vi "FGV CalGas.vi"(6 "Aktionen":T8, 7 "Analysator Auswahl":T1 {"Analysator Auswahl 12" items=["----"=100, "FT-IR"=0, "TEST"=1]; "Analysator Auswahl 11" items=["----"=100, "FT-IR"=0, "TEST"=1]; "Analysator Auswahl 10" items=["----"=100, "FT-IR"=0, "TEST"=1]; "Analysator Auswahl 9" items=["----"=100, "FT-IR"=0, "TEST"=1]; "Analysator Auswahl 8" items=["----"=100, "FT-IR"=0, "TEST"=1]; "Analysator Auswahl 7" items=["----"=100, "FT-IR"=0, "TEST"=1]; "Analysator Auswahl 6" items=["----"=100, "FT-IR"=0, "TEST"=1]; "Analysator Auswahl 5" items=["----"=100, "FT-IR"=0, "TEST"=1]; "Analysator Auswahl 4" items=["----"=100, "FT-IR"=0, "TEST"=1]; "Analysator Auswahl 3" items=["----"=100, "FT-IR"=0, "TEST"=1]; "Analysator Auswahl 2" items=["----"=100, "FT-IR"=0, "TEST"=1]; "Analysator Auswahl" items=["----"=100, "FT-IR"=0, "PMA"=1]}, 10 "Aufschaltung CalGas":T4 {"Kalibriergas" items=["Stickstoff", "---", "---", "NOx lo", "NOx hi", "---", "CO2", "CO", "---", "O2", "---", "HC", "---"]}, 11 "Def.CalGas neu":T9 {"Messbereiche"."Messbereich 12" items=["0-100ppm", "0-1000ppm", "0-5000ppm"]; "Messbereiche"."Messbereich 11" items=["0-100ppm", "0-1000ppm", "0-5000ppm"]; "Messbereiche"."Messbereich 10" items=["0-100ppm", "0-1000ppm", "0-5000ppm"]; "Messbereiche"."Messbereich 9" items=["0-100ppm", "0-1000ppm", "0-5000ppm"]; "Messbereiche"."Messbereich 8" items=["0-100ppm", "0-1000ppm", "0-5000ppm"]; "Messbereiche"."Messbereich 7" items=["0-100ppm", "0-1000ppm", "0-5000ppm"]; "Messbereiche"."Messbereich 6" items=["0-100ppm", "0-1000ppm", "0-5000ppm"]; "Messbereiche"."Messbereich 5" items=["0-100ppm", "0-1000ppm", "0-5000ppm"]; "Messbereiche"."Messbereich 4" items=["0-100ppm", "0-1000ppm", "0-5000ppm"]; "Messbereiche"."Messbereich 3" items=["0-100ppm", "0-1000ppm", "0-5000ppm"]; "Messbereiche"."Messbereich 2" items=["0-100ppm", "0-1000ppm", "0-5000ppm"]; "Messbereiche"."Messbereich 1" items=["0-100ppm", "0-1000ppm", "0-5000ppm"]; "Einheit"."Einheit 12" items=["ppm", "%"]; "Einheit"."Einheit 11" items=["ppm", "%"]; "Einheit"."Einheit 10" items=["ppm", "%"]; "Einheit"."Einheit 9" items=["ppm", "%"]; "Einheit"."Einheit 8" items=["ppm", "%"]; "Einheit"."Einheit 7" items=["ppm", "%"]; "Einheit"."Einheit 6" items=["ppm", "%"]; "Einheit"."Einheit 5" items=["ppm", "%"]; "Einheit"."Einheit 4" items=["ppm", "%"]; "Einheit"."Einheit 3" items=["ppm", "%"]; "Einheit"."Einheit 2" items=["ppm", "%"]; "Einheit"."Einheit 1" items=["ppm", "%"]; "Werte 2"."Konzentration 12" format="%#_5g"; "Werte 2"."Konzentration 11" format="%#_5g"; "Werte 2"."Konzentration 10" format="%#_5g"; "Werte 2"."Konzentration 9" format="%#_5g"; "Werte 2"."Konzentration 8" format="%#_5g"; "Werte 2"."Konzentration 7" format="%#_5g"; "Werte 2"."Konzentration 6" format="%#_5g"; "Werte 2"."Konzentration 5" format="%#_5g"; "Werte 2"."Konzentration 4" format="%#_5g"; "Werte 2"."Konzentration 3" format="%#_5g"; "Werte 2"."Konzentration 2" format="%#_5g"; "Werte 2"."Konzentration 1" format="%#_5g"; "Werte"."Konzentration 12" format="%#_5g"; "Werte"."Konzentration 11" format="%#_5g"; "Werte"."Konzentration 10" format="%#_5g"; "Werte"."Konzentration 9" format="%#_5g"; "Werte"."Konzentration 8" format="%#_5g"; "Werte"."Konzentration 7" format="%#_5g"; "Werte"."Konzentration 6" format="%#_5g"; "Werte"."Konzentration 5" format="%#_5g"; "Werte"."Konzentration 4" format="%#_5g"; "Werte"."Konzentration 3" format="%#_5g"; "Werte"."Konzentration 2" format="%#_5g"; "Werte"."Konzentration 1" format="%#_5g"}) -> (0 "Konzentration 2":T3 format="%#_5g", 1 "Konzentration 1":T3 format="%#_5g", 2 "Aufschaltung CalGas":T4, 3 "Def.CalGas":T9 {"Messbereiche"."Messbereich 12" items=["0-100ppm", "0-1000ppm", "0-5000ppm"]; "Messbereiche"."Messbereich 11" items=["0-100ppm", "0-1000ppm", "0-5000ppm"]; "Messbereiche"."Messbereich 10" items=["0-100ppm", "0-1000ppm", "0-5000ppm"]; "Messbereiche"."Messbereich 9" items=["0-100ppm", "0-1000ppm", "0-5000ppm"]; "Messbereiche"."Messbereich 8" items=["0-100ppm", "0-1000ppm", "0-5000ppm"]; "Messbereiche"."Messbereich 7" items=["0-100ppm", "0-1000ppm", "0-5000ppm"]; "Messbereiche"."Messbereich 6" items=["0-100ppm", "0-1000ppm", "0-5000ppm"]; "Messbereiche"."Messbereich 5" items=["0-100ppm", "0-1000ppm", "0-5000ppm"]; "Messbereiche"."Messbereich 4" items=["0-100ppm", "0-1000ppm", "0-5000ppm"]; "Messbereiche"."Messbereich 3" items=["0-100ppm", "0-1000ppm", "0-5000ppm"]; "Messbereiche"."Messbereich 2" items=["0-100ppm", "0-1000ppm", "0-5000ppm"]; "Messbereiche"."Messbereich 1" items=["0-100ppm", "0-1000ppm", "0-5000ppm"]; "Einheit"."Einheit 12" items=["ppm", "%"]; "Einheit"."Einheit 11" items=["ppm", "%"]; "Einheit"."Einheit 10" items=["ppm", "%"]; "Einheit"."Einheit 9" items=["ppm", "%"]; "Einheit"."Einheit 8" items=["ppm", "%"]; "Einheit"."Einheit 7" items=["ppm", "%"]; "Einheit"."Einheit 6" items=["ppm", "%"]; "Einheit"."Einheit 5" items=["ppm", "%"]; "Einheit"."Einheit 4" items=["ppm", "%"]; "Einheit"."Einheit 3" items=["ppm", "%"]; "Einheit"."Einheit 2" items=["ppm", "%"]; "Einheit"."Einheit 1" items=["ppm", "%"]; "Werte 2"."Konzentration 12" format="%#_5g"; "Werte 2"."Konzentration 11" format="%#_5g"; "Werte 2"."Konzentration 10" format="%#_5g"; "Werte 2"."Konzentration 9" format="%#_5g"; "Werte 2"."Konzentration 8" format="%#_5g"; "Werte 2"."Konzentration 7" format="%#_5g"; "Werte 2"."Konzentration 6" format="%#_5g"; "Werte 2"."Konzentration 5" format="%#_5g"; "Werte 2"."Konzentration 4" format="%#_5g"; "Werte 2"."Konzentration 3" format="%#_5g"; "Werte 2"."Konzentration 2" format="%#_5g"; "Werte 2"."Konzentration 1" format="%#_5g"; "Werte"."Konzentration 12" format="%#_5g"; "Werte"."Konzentration 11" format="%#_5g"; "Werte"."Konzentration 10" format="%#_5g"; "Werte"."Konzentration 9" format="%#_5g"; "Werte"."Konzentration 8" format="%#_5g"; "Werte"."Konzentration 7" format="%#_5g"; "Werte"."Konzentration 6" format="%#_5g"; "Werte"."Konzentration 5" format="%#_5g"; "Werte"."Konzentration 4" format="%#_5g"; "Werte"."Konzentration 3" format="%#_5g"; "Werte"."Konzentration 2" format="%#_5g"; "Werte"."Konzentration 1" format="%#_5g"}, 5 "Analysator Auswahl":T1 {"Analysator Auswahl 12" items=["----"=100, "FT-IR"=0, "TEST"=1]; "Analysator Auswahl 11" items=["----"=100, "FT-IR"=0, "TEST"=1]; "Analysator Auswahl 10" items=["----"=100, "FT-IR"=0, "TEST"=1]; "Analysator Auswahl 9" items=["----"=100, "FT-IR"=0, "TEST"=1]; "Analysator Auswahl 8" items=["----"=100, "FT-IR"=0, "TEST"=1]; "Analysator Auswahl 7" items=["----"=100, "FT-IR"=0, "TEST"=1]; "Analysator Auswahl 6" items=["----"=100, "FT-IR"=0, "TEST"=1]; "Analysator Auswahl 5" items=["----"=100, "FT-IR"=0, "TEST"=1]; "Analysator Auswahl 4" items=["----"=100, "FT-IR"=0, "TEST"=1]; "Analysator Auswahl 3" items=["----"=100, "FT-IR"=0, "TEST"=1]; "Analysator Auswahl 2" items=["----"=100, "FT-IR"=0, "TEST"=1]; "Analysator Auswahl" items=["----"=100, "FT-IR"=0, "PMA"=1]})   [LabVIEW 2020, in "CalGas Aufschaltung.lvlib"]
uses:
  CalGas Aufschaltung.lvlib
  Definition CalGas Anzeige.ctl
  CalGas-Namen.ctl
  Visualisierungs Elemente/String - Eingabefeld.ctl
  CalGas-Werte.ctl
  Visualisierungs Elemente/Zahlen-Eingabefeld.ctl
  CalGas-Einheit.ctl
  Visualisierungs Elemente/Auswahlfeld.ctl
  CalGas-Messbereiche.ctl
  FGV CalGas Aktionen.ctl
  Aufschaltung CalGas.ctl
  Auswahl Aufschaltpunkt.ctl
  Auswahl Analysator.ctl
  Cluster Auswahl Analysator.ctl
  Analysator Auswahl.ctl
  Analysator Definition/FGV Analysator Definition Aktionen.ctl
  Allgemein/allgemeine Sub-VIs.lvlib
  Analysator Definition/Analysator Definition.lvlib
panel:
  # "Span 1"
  # "Span 2"
  # "Span 3"
  # "Span 4"
  # "Span 5"
  # "Span 6"
  # "Span 7"
  # "Span 8"
  # "Span 9"
  # "Span 10"
  # "Span 11"
  # "Span 12"
  # "Span 1"
  # "Span 2"
  # "Span 3"
  # "Span 4"
  # "Span 5"
  # "Span 6"
  # "Span 7"
  # "Span 8"
  # "Span 9"
  # "Span 10"
  # "Span 11"
  # "Span 12"
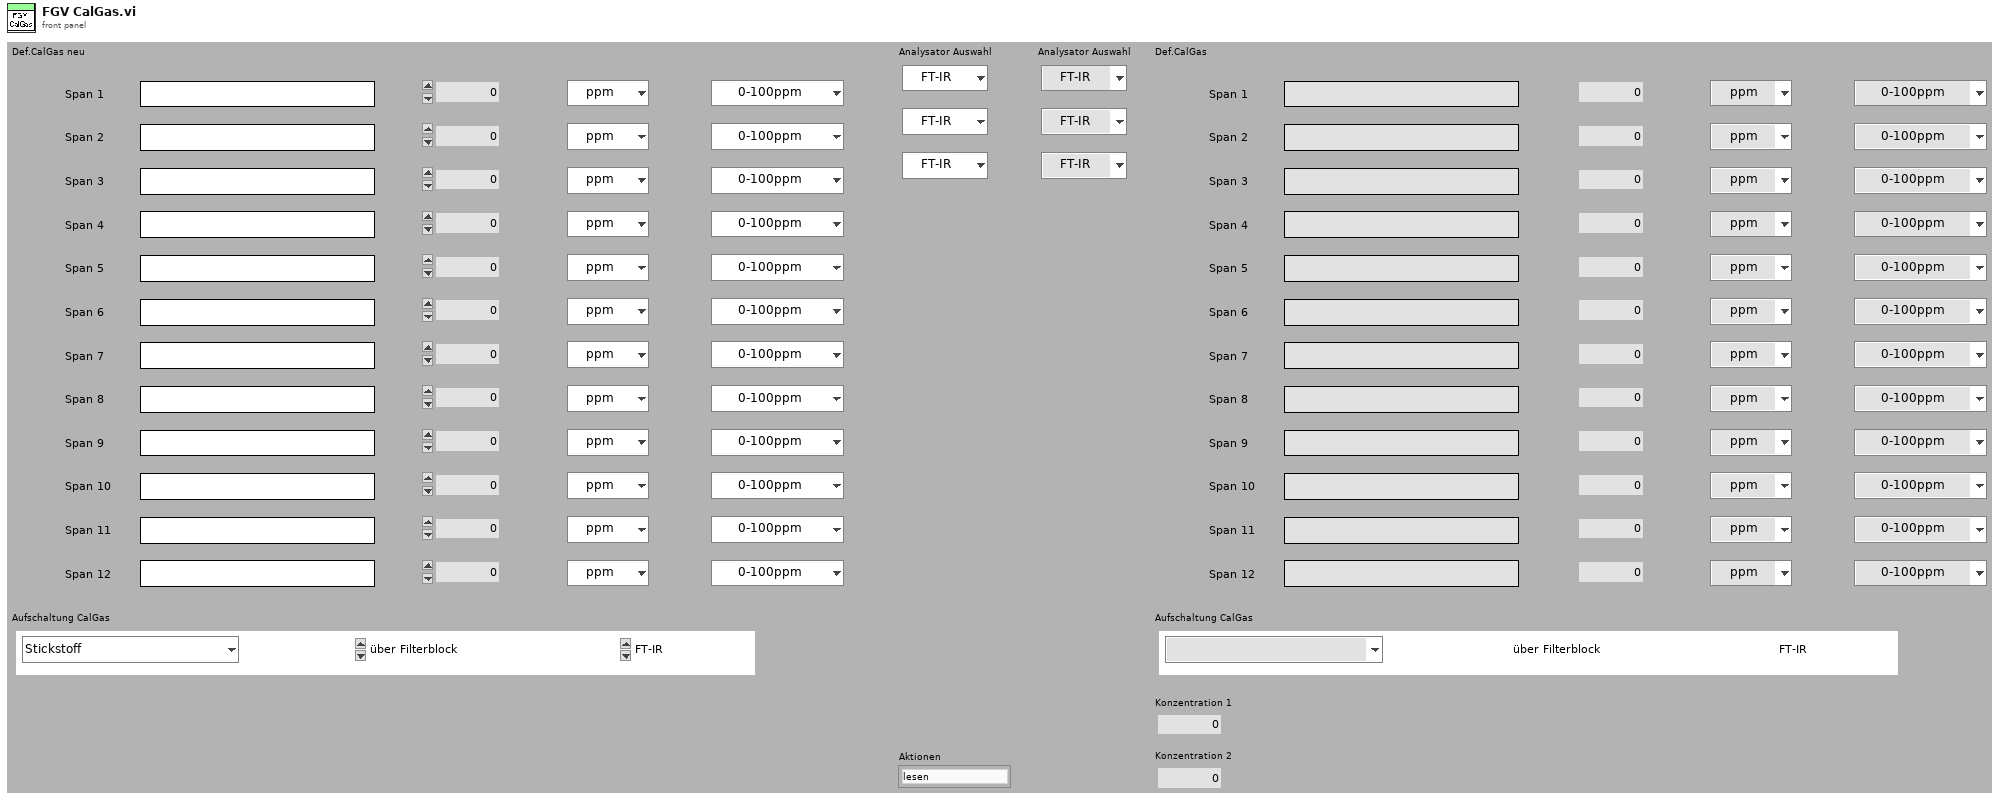
[diagram p1: front panel]
types:
  T1 = typedef "CalGas Aufschaltung.lvlib/Cluster Auswahl Analysator.ctl" = cluster{"Analysator Auswahl":T2, "Analysator Auswahl 2":T2, "Analysator Auswahl 3":T2, "Analysator Auswahl 4":T2, "Analysator Auswahl 5":T2, "Analysator Auswahl 6":T2, "Analysator Auswahl 7":T2, "Analysator Auswahl 8":T2, "Analysator Auswahl 9":T2, "Analysator Auswahl 10":T2, "Analysator Auswahl 11":T2, "Analysator Auswahl 12":T2}
  T2 = typedef "CalGas Aufschaltung.lvlib/Analysator Auswahl.ctl" = u16
  T3 = typedef "Zahlen-Eingabefeld.ctl" = sgl
  T4 = typedef "CalGas Aufschaltung.lvlib/Aufschaltung CalGas.ctl" = cluster{"Kalibriergas":T5, "Aufschaltpunkt":T6, "Analysator":T7}
  T5 = typedef "Auswahlfeld.ctl" = u16
  T6 = typedef "CalGas Aufschaltung.lvlib/Auswahl Aufschaltpunkt.ctl" = enum16{"über Filterblock", "Analysator direkt", "über PNS", "Entnahme", "Gasdivider"}
  T7 = typedef "CalGas Aufschaltung.lvlib/Auswahl Analysator.ctl" = enum16{"FT-IR", "FID", "PMA", "PMA/FID/FT-IR"}
  T8 = typedef "CalGas Aufschaltung.lvlib/FGV CalGas Aktionen.ctl" = enum16{"lesen", "Analysator Auswahl", "Def.CalGas", "Aufschaltung CalGas", "laden", "speichern", "KAL extrahieren"}
  T9 = typedef "CalGas Aufschaltung.lvlib/Definition CalGas Anzeige.ctl" = cluster{"Namen":T10, "Werte":T12, "Werte 2":T12, "Einheit":T13, "Messbereiche":T14}
  T10 = typedef "CalGas Aufschaltung.lvlib/CalGas-Namen.ctl" = cluster{"Name":T11, "Name 2":T11, "Name 3":T11, "Name 4":T11, "Name 5":T11, "Name 6":T11, "Name 7":T11, "Name 8":T11, "Name 9":T11, "Name 10":T11, "Name 11":T11, "Name 12":T11}
  T11 = typedef "String - Eingabefeld.ctl" = string
  T12 = typedef "CalGas Aufschaltung.lvlib/CalGas-Werte.ctl" = cluster{"Konzentration 1":T3, "Konzentration 2":T3, "Konzentration 3":T3, "Konzentration 4":T3, "Konzentration 5":T3, "Konzentration 6":T3, "Konzentration 7":T3, "Konzentration 8":T3, "Konzentration 9":T3, "Konzentration 10":T3, "Konzentration 11":T3, "Konzentration 12":T3}
  T13 = typedef "CalGas Aufschaltung.lvlib/CalGas-Einheit.ctl" = cluster{"Einheit 1":T5, "Einheit 2":T5, "Einheit 3":T5, "Einheit 4":T5, "Einheit 5":T5, "Einheit 6":T5, "Einheit 7":T5, "Einheit 8":T5, "Einheit 9":T5, "Einheit 10":T5, "Einheit 11":T5, "Einheit 12":T5}
  T14 = typedef "CalGas Aufschaltung.lvlib/CalGas-Messbereiche.ctl" = cluster{"Messbereich 1":T5, "Messbereich 2":T5, "Messbereich 3":T5, "Messbereich 4":T5, "Messbereich 5":T5, "Messbereich 6":T5, "Messbereich 7":T5, "Messbereich 8":T5, "Messbereich 9":T5, "Messbereich 10":T5, "Messbereich 11":T5, "Messbereich 12":T5}
  T15 = typedef "Analysator Definition.lvlib/FGV Analysator Definition Aktionen.ctl" = enum16{"lesen", "MB setzen", "MB KAL setzen", "laden"}
  T16 = cluster{"Def.CalGas neu":T9, "Aufschaltung CalGas":T4, "Analysator Auswahl":T1}
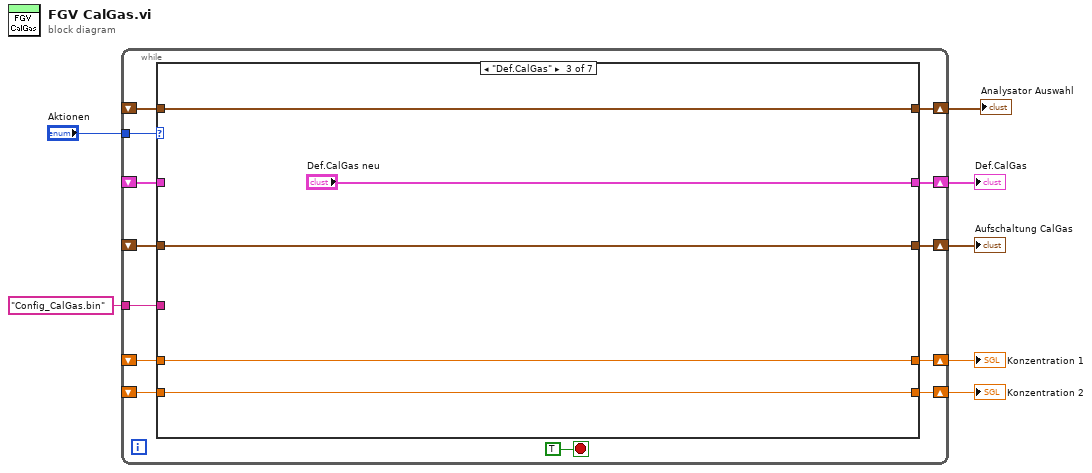
[diagram p0: block diagram]
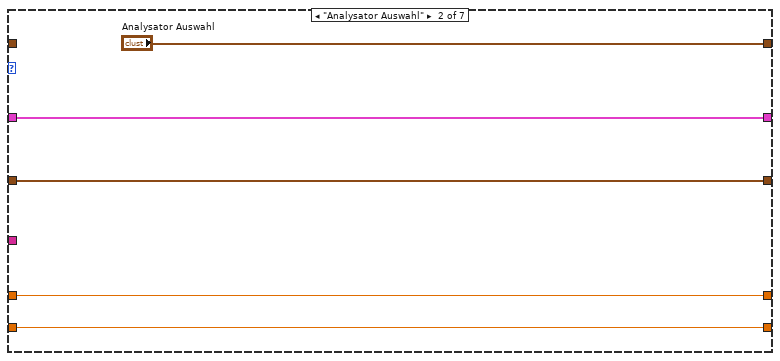
[diagram p3: hidden frame]
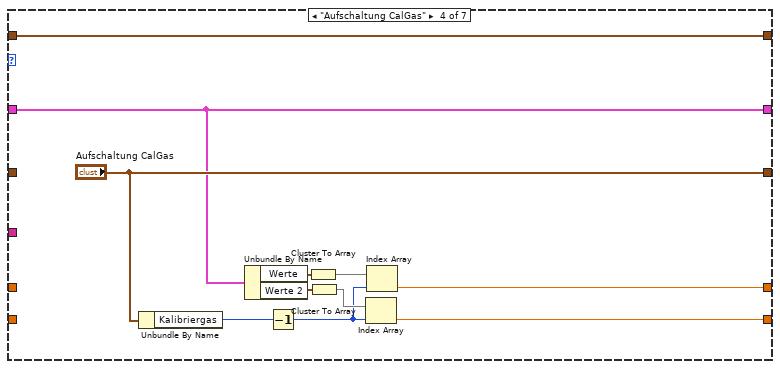
[diagram p4: hidden frame]
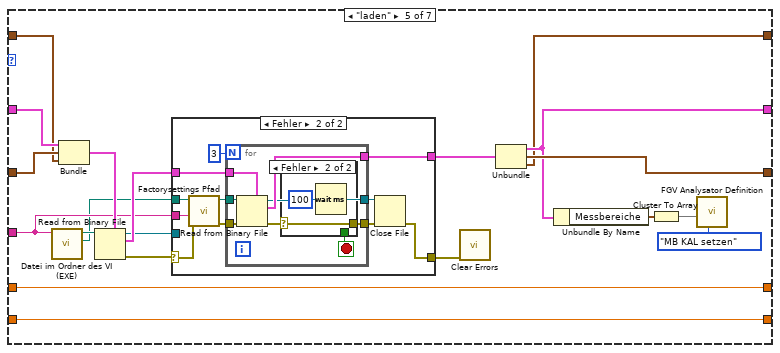
[diagram p5: hidden frame]
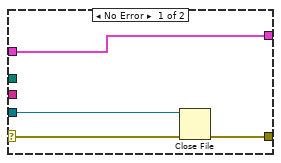
[diagram p6: hidden frame]
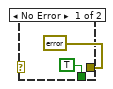
[diagram p7: hidden frame]
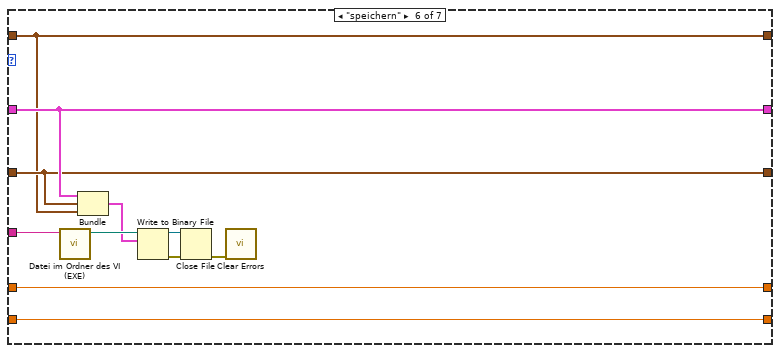
[diagram p8: hidden frame]
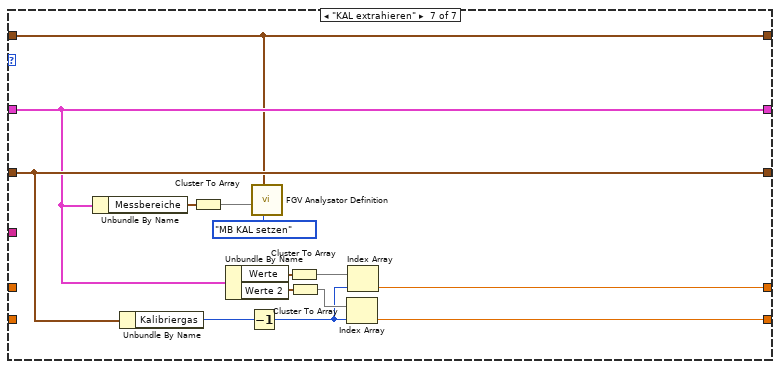
[diagram p9: hidden frame]
diagram:
  n1 = while {
    tunnel: "Aktionen" -> [w19]
    shift-right: [w18] -> w4
    shift-left: _ -> [w17]
    shift-right: [w16] -> w6
    shift-left: _ -> [w15]
    tunnel: "Config_CalGas.bin" ("Dateiname") -> [w14]
    shift-right: [w12] -> w3
    shift-left: _ -> [w11]
    shift-right: [w13] -> w2
    shift-left: _ -> [w10]
    shift-right: [w9] -> w1
    shift-left: _ -> [w8]
    stop <- TRUE stop-if-true
    n2 = case shown="\"Def.CalGas\"" w19 {
      tunnel: [w25 w30 "Def.CalGas neu" w44 w61 w101 w109] -> w18
      tunnel: w17 -> [w25 w30 _ w44 w64 w101 w109]
      tunnel: [w24 w29 w35 "Aufschaltung CalGas" w63 w100 w110] -> w16
      tunnel: w15 -> [w24 w29 w35 _ w66 w100 w110]
      tunnel: w14 -> [_ _ _ _ w50 w103 _]
      tunnel: [w22 w27 w32 w40 w59 w98 w108] -> w13
      tunnel: [w23 w28 w33 w39 w60 w99 w111] -> w12
      tunnel: w11 -> [w23 w28 w33 _ w60 w99 _]
      tunnel: w10 -> [w22 w27 w32 _ w59 w98 _]
      tunnel: [w21 "Analysator Auswahl" w31 w36 w55 w94 w105] -> w9
      tunnel: w8 -> [w21 _ w31 w36 w56 w94 w105]
      frame "lesen", Default {
      }
      frame "Analysator Auswahl" {
      }
      frame "Def.CalGas" {
      }
      frame "Aufschaltung CalGas" {
        n3 = Unbundle By Name("Aufschaltung CalGas") -> ("Kalibriergas"=w38:T5)
        n4 = Unbundle By Name(w44) -> ("Werte"=w46:T12, "Werte 2"=w42:T12)
        n5 = Decrement(x=w38) -> (x-1=w37:T5)
        n6 = Cluster To Array(cluster=w46) -> (array=w43:T3[])
        n7 = Cluster To Array(cluster=w42) -> (array=w41:T3[])
        n8 = Index Array(array=w41, index=w37) -> (element=w40:T3)
        n9 = Index Array(array=w43, index=w37) -> (element=w39:T3)
      }
      frame "laden" {
        n10 = call "Datei im Ordner des VI (EXE).vi"("Dateiname"=w50) -> ("Ordner des Haupt-VIs"=w47:path, "Dateipfad im Ordner des Haupt-VIs"=w51:path)  [unwired: 8 in, 1 out]
        n11 = Bundle("Def.CalGas neu"=w64, "Aufschaltung CalGas"=w66, "Analysator Auswahl"=w56) -> (w65:T16)  [unwired: 1 in]
        n12 = Read from Binary File(5:w65, 11:w51) -> (0:w48:errorcluster, 2:w53:T16, 3:w49:refnum<file>)  [unwired: 1 in, 4 out]
        n13 = case shown="Fehler" w48 {
          selector: w48 -> [w69 w73]
          tunnel: w53 -> [w70 w76]
          tunnel: [w70 w80] -> w52
          tunnel: [w67 w78] -> w54
          tunnel: w49 -> [w68 _]
          tunnel: w47 -> [_ w72]
          tunnel: w50 -> [_ w71]
          frame No Error {
            n14 = Close File(refnum=w68, error in=w69) -> (error out=w67:errorcluster)  [unwired: 1 out]
          }
          frame Error {
            n15 = call "Factorysettings Pfad.vi"("error in (no error)"=w73, "Dateiname"=w71, "Ordner des Haupt-VIs"=w72) -> ("error out"=w74:errorcluster, "Pfad Factorysettings"=w75:path)  [unwired: 7 in]
            n16 = for {
              N: 3 -> [_]
              tunnel: w74 -> [w87]
              tunnel: w75 -> [w86]
              tunnel: [w85] -> w80
              tunnel: [w84] -> w79
              tunnel: [w83] -> w77
              tunnel: w76 -> [w82]
              stop <- w88 stop-if-true
              n17 = Read from Binary File(5:w82, 8:w87, 11:w86) -> (0:w89:errorcluster, 2:w85:T16, 3:w83:refnum<file>)  [unwired: 3 in, 1 out]
              n18 = case shown="Fehler" w89 {
                selector: w89 -> [_ w92]
                tunnel: [TRUE _] -> w88
                tunnel: [errorcluster {"status"=FALSE, "code"=0, "source"=""} ("error IO") w92] -> w84
                frame No Error {
                }
                frame Error {
                  n19 = Wait (ms)(milliseconds to wait=u32 100 ("Zu wartende ms")) -> ()  [unwired: 1 out]
                }
              }
            }
            n20 = Close File(refnum=w77, error in=w79) -> (error out=w78:errorcluster)  [unwired: 1 out]
          }
        }
        n21 = call <vilib>:"Clear Errors.vi"("error in (no error)"=w54) -> ()  [unwired: 5 in, 2 out]
        n22 = Unbundle(w52) -> ("Def.CalGas neu"=w61:T9, "Aufschaltung CalGas"=w63:T4, "Analysator Auswahl"=w55:T1)
        n23 = Unbundle By Name(w61) -> ("Messbereiche"=w62:T14)
        n24 = Cluster To Array(cluster=w62) -> (array=w57:T5[])
        n25 = call "FGV Analysator Definition.vi"("Aktionen"=FGV_Analysator_Definition_Aktionen."MB KAL setzen", "Messbereiche KAL"=w57) -> ()  [unwired: 5 in, 5 out]
      }
      frame "speichern" {
        n26 = call "Datei im Ordner des VI (EXE).vi"("Dateiname"=w103) -> ("Dateipfad im Ordner des Haupt-VIs"=w104:path)  [unwired: 8 in, 2 out]
        n27 = Bundle("Def.CalGas neu"=w101, "Aufschaltung CalGas"=w100, "Analysator Auswahl"=w94) -> (w102:T16)  [unwired: 1 in]
        n28 = Write to Binary File(file (use dialog)=w104, data=w102) -> (refnum out=w96:refnum<file>, error out=w97:errorcluster)  [unwired: 2 in, 3 out]
        n29 = Close File(refnum=w96, error in=w97) -> (error out=w95:errorcluster)  [unwired: 1 out]
        n30 = call <vilib>:"Clear Errors.vi"("error in (no error)"=w95) -> ()  [unwired: 5 in, 2 out]
      }
      frame "KAL extrahieren" {
        n31 = Unbundle By Name(w109) -> ("Messbereiche"=w118:T14)
        n32 = Unbundle By Name(w110) -> ("Kalibriergas"=w113:T5)
        n33 = Cluster To Array(cluster=w118) -> (array=w106:T5[])
        n34 = Unbundle By Name(w109) -> ("Werte"=w117:T12, "Werte 2"=w115:T12)
        n35 = Decrement(x=w113) -> (x-1=w112:T5)
        n36 = call "FGV Analysator Definition.vi"("Aktionen"=FGV_Analysator_Definition_Aktionen."MB KAL setzen", "Analysator Auswahl"=w105, "Messbereiche KAL"=w106) -> ()  [unwired: 4 in, 5 out]
        n37 = Cluster To Array(cluster=w117) -> (array=w116:T3[])
        n38 = Cluster To Array(cluster=w115) -> (array=w114:T3[])
        n39 = Index Array(array=w114, index=w112) -> (element=w108:T3)
        n40 = Index Array(array=w116, index=w112) -> (element=w111:T3)
      }
    }
  }
  "Def.CalGas" <- w4
  "Aufschaltung CalGas" <- w6
  "Konzentration 1" <- w3
  "Konzentration 2" <- w2
  "Analysator Auswahl" <- w1
